vi "Send and Receive Message.vi"(6 "timeout in ms (-1)":i32=-1, 8 "error in":errorcluster, 9 "Message in":refnum<class "Abstract Message.lvclass">, 11 "Consumer Information":T1) -> (0 "error out":errorcluster, 1 "Message out":refnum<class "Abstract Message.lvclass">, 4 "timed out?":bool)   [LabVIEW 2020, in "Messaging.lvlib" / "Abstract Producer.lvclass"]
uses:
  Abstract Producer.lvclass
  Message Queue/Abstract Message Queue/Abstract Message Queue.lvclass
  Consumer Information.ctl
  Message/Abstract Message/Abstract Message.lvclass
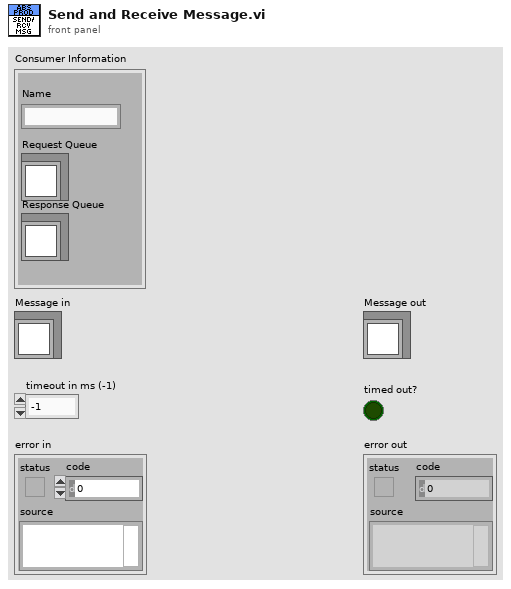
[diagram p1: front panel]
types:
  T1 = typedef "Messaging.lvlib/Abstract Producer.lvclass/Consumer Information.ctl" = cluster{"Name":string, "Request Queue":refnum<class "Abstract Message Queue.lvclass">, "Response Queue":refnum<class "Abstract Message Queue.lvclass">}
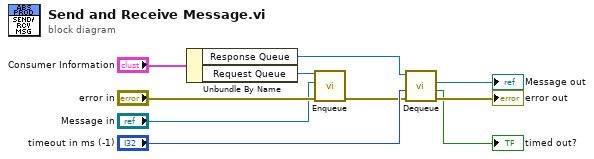
[diagram p0: block diagram]
diagram:
  n1 = Unbundle By Name("Consumer Information") -> ("Response Queue"=w1:refnum<class "Abstract Message Queue.lvclass">, "Request Queue"=w3:refnum<class "Abstract Message Queue.lvclass">)
  n2 = call-dynamic "Enqueue.vi"("error in (no error)"="error in", "Message in"="Message in", "Abstract Message Queue in"=w3) -> ("error out"=w2:errorcluster)  [unwired: 7 in, 1 out]
  n3 = call-dynamic "Dequeue.vi"("error in (no error)"=w2, "timeout in ms (-1)"="timeout in ms (-1)", "Abstract Message Queue in"=w1) -> ("error out"=→"error out":errorcluster, "timed out?"=→"timed out?":bool, "Message out"=→"Message out":refnum<class "Abstract Message.lvclass">)  [unwired: 5 in, 1 out]
